vi "FFT 1D real 2 cplx (poly).vi"   [LabVIEW 2020, in "FFTWDLL.lvlib"]
doc: "1D FFT with real input and cplx output. Combines all FFTW steps (allocations, planing, freeing memory). May not be effective for repeated calls!"
uses:
  FFTWDLL.lvlib
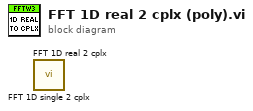
[diagram p0: block diagram]
diagram:
  n1 = call "FFT 1D single 2 cplx.vi"() -> ()  [unwired: 8 in, 4 out]
  n2 = call "FFT 1D real 2 cplx.vi"() -> ()  [unwired: 8 in, 4 out]
